vi "ORP滴定曲线.vi"(8 "error in (no error)":errorcluster) -> (0 "error out":errorcluster, 3 "输出数组":u16[](array[numeric]))   [LabVIEW 2016, in "一代CodMn.lvlib"]
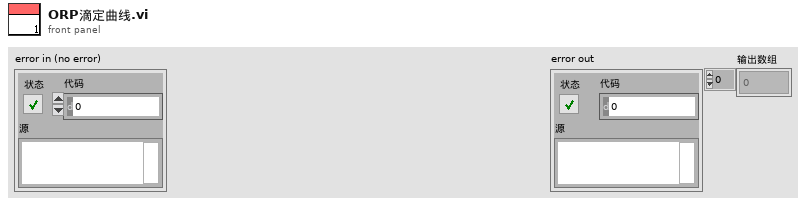
[diagram p1: front panel]
types:
  T1 = enum16{"open", "close", "readHR", "writeHR", "readCoil", "writeCoil"}
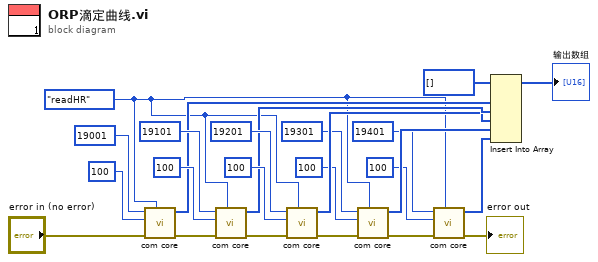
[diagram p0: block diagram]
diagram:
  w1 = T1."readHR" ("功能")
  n1 = call "com core.vi"("功能"=w1, "error in (no error)"="error in (no error)", "quantity"=u16 100, "starting address"=u16 19001) -> ("error out"=w22:errorcluster, "Registers"=w15:u16[])  [unwired: 5 in, 1 out]
  n2 = call "com core.vi"("功能"=w1, "error in (no error)"=w22, "quantity"=u16 100, "starting address"=u16 19101) -> ("error out"=w21:errorcluster, "Registers"=w14:u16[])  [unwired: 5 in, 1 out]
  n3 = call "com core.vi"("功能"=w1, "error in (no error)"=w21, "quantity"=u16 100, "starting address"=u16 19201) -> ("error out"=w9:errorcluster, "Registers"=w13:u16[])  [unwired: 5 in, 1 out]
  n4 = call "com core.vi"("功能"=w1, "error in (no error)"=w9, "quantity"=u16 100, "starting address"=u16 19301) -> ("error out"=w10:errorcluster, "Registers"=w7:u16[])  [unwired: 5 in, 1 out]
  n5 = call "com core.vi"("功能"=w1, "error in (no error)"=w10, "quantity"=u16 100, "starting address"=u16 19401) -> ("error out"=→"error out":errorcluster, "Registers"=w6:u16[])  [unwired: 5 in, 1 out]
  n6 = Insert Into Array(array=u16[] [] ("数组"), new element #1=w15, new element #2=w14, new element #3=w13, new element #4=w7, new element #5=w6) -> (→"输出数组":u16[])  [unwired: 1 in]
